vi "POLL BIAS.vi"(8 "error in (no error)":errorcluster, 9 "element":T1 {"Avoid zero threshold (V)" format="%#_13g"}, 10 "ScanQ in":refnum<queue>, 11 "Queue in":refnum<queue>) -> (0 "error out":errorcluster, 2 "ScanQ out":refnum<queue>, 3 "Queue out":refnum<queue>)   [LabVIEW 2025]
uses:
  Desktop/STM-Auto-Project/QMH CTLS/Scan_Params (QMH).ctl
  TEMP_SWEEPER.ctl
  <userlib>/Nanonis Prog Interface V5e/Nanonis Prog Interface.lvlib
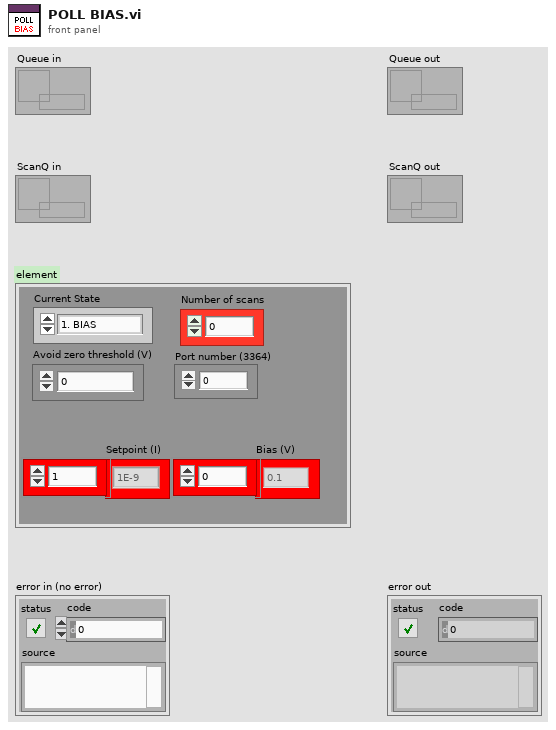
[diagram p1: front panel]
types:
  T1 = typedef "Scan_Params (QMH).ctl" = cluster{"Setpoint (I)":dbl[], "Bias (V)":dbl[], "Number of scans":u8, "Port number (3364)":u32, "Avoid zero threshold (V)":dbl, "Current State":enum16{"1. BIAS", "2. INIT_SCAN", "3. SCAN_IDLE", "4. INTER_SCAN", "5. NEW_COORDS_&_FRAME", "6. FINAL_SCAN", "7. POLL BIAS ", "8. Z-CONT.", "9. STOP"}}
  T2 = enum16{"1. BIAS", "2. INIT_SCAN", "3. SCAN_IDLE", "4. INTER_SCAN", "5. NEW_COORDS_&_FRAME", "6. FINAL_SCAN", "7. POLL BIAS ", "8. Z-CONT.", "9. STOP"}
  T3 = enum16{"SET TEMP", "SWEEP IDLE", "NEXT TEMP", "SWEEP DONE"}
  T4 = typedef "TEMP_SWEEPER.ctl" = cluster{"Temps(K)":dbl[], "Sweep States":enum16{"SET TEMP", "SWEEP IDLE", "NEXT TEMP", "SWEEP DONE"}}
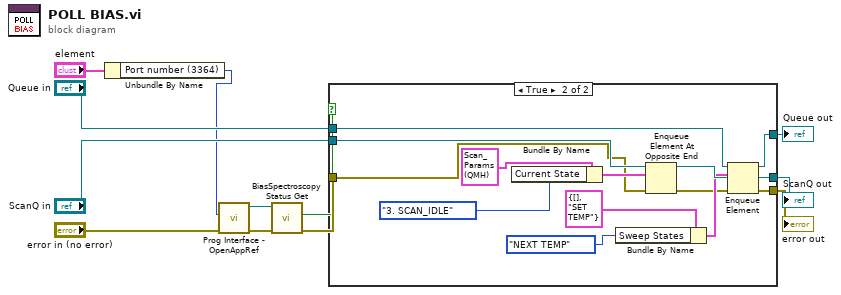
[diagram p0: block diagram]
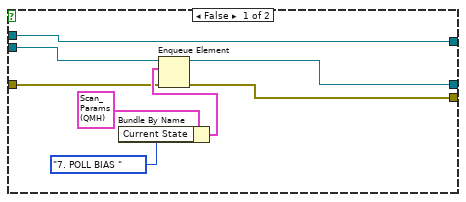
[diagram p2: hidden frame]
diagram:
  n1 = Unbundle By Name("element") -> ("Port number (3364)"=w1:u32)
  n2 = call <userlib>:"Prog Interface - OpenAppRef.vi"("Error in (no error)"="error in (no error)", "Port number (3364)"=w1) -> ("Error out"=w4:errorcluster, "Application reference"=w3:refnum<vi>)  [unwired: 4 in]
  n3 = call <userlib>:"BiasSpectroscopy Status Get.vi"("Error in (no error)"=w4, "Application ref in"=w3) -> ("Error out"=w11:errorcluster, "Running?"=w5:bool)  [unwired: 5 in, 1 out]
  n4 = case shown="True" w5 {
    tunnel: "ScanQ in" -> [w20 w33]
    tunnel: [w17 w30] -> w7
    tunnel: "Queue in" -> [w14 w29]
    tunnel: [w14 w28] -> w9
    tunnel: [w15 w24] -> w10
    tunnel: w11 -> [w16 w23]
    frame False {
      n5 = Bundle By Name(cluster=T1 {"Setpoint (I)"=[], "Bias (V)"=[], "Number of scans"=1, "Port number (3364)"=3364, "Avoid zero threshold (V)"=0.004999999888241291, "Current State"=enum."1. BIAS"} ("element"), "Current State"=T2."7. POLL BIAS ") -> (w18:T1)
      n6 = Enqueue Element(queue=w20, element=w18, error in (no error)=w16) -> (queue out=w17:refnum<queue>, error out=w15:errorcluster)  [unwired: 1 in, 1 out]
    }
    frame True {
      n7 = Bundle By Name(cluster=T1 {"Setpoint (I)"=[], "Bias (V)"=[], "Number of scans"=1, "Port number (3364)"=3364, "Avoid zero threshold (V)"=0.004999999888241291, "Current State"=enum."1. BIAS"} ("element"), "Current State"=T2."3. SCAN_IDLE") -> (w31:T1)
      n8 = Bundle By Name(cluster=T4 {"Temps(K)"=[], "Sweep States"=enum."SET TEMP"} ("Temp and Field Range"), "Sweep States"=T3."NEXT TEMP") -> (w26:T4)
      n9 = Enqueue Element At Opposite End(queue=w33, element=w31, error in (no error)=w23) -> (queue out=w30:refnum<queue>, error out=w25:errorcluster)  [unwired: 1 in, 1 out]
      n10 = Enqueue Element(queue=w29, element=w26, error in (no error)=w25) -> (queue out=w28:refnum<queue>, error out=w24:errorcluster)  [unwired: 1 in, 1 out]
    }
  }
  "error out" <- w10
  "Queue out" <- w9
  "ScanQ out" <- w7
